vi "Check Status (No Objects).vi"(8 "error in (no error)":errorcluster, 11 "Cluster In":T3={"helium"={"fastHe?"=FALSE, "slowHe?"=FALSE, "fillHe?"=FALSE, "lowHe?"=FALSE}, "nitrogen"={"fillN?"=FALSE, "lowN?"=FALSE}, "Shutdown"=FALSE, "Cryogen Levels"=[], "IO Info"={"Address"={"Com Port"=1, "ISOBUS Address"=5, "GPIB Address"=24, "Communication"=enum."ISOBUS"}, "ILM Name"="", "Display Channel"=[]}} {"Cryogen Levels" min=-1.0 max=100.0 scale=0.0..100.0}) -> (0 "error out":errorcluster, 1 "Status":string, 2 "On?":bool, 3 "Cluster Out":T3={"helium"={"fastHe?"=FALSE, "slowHe?"=FALSE, "fillHe?"=FALSE, "lowHe?"=FALSE}, "nitrogen"={"fillN?"=FALSE, "lowN?"=FALSE}, "Shutdown"=FALSE, "Cryogen Levels"=[], "IO Info"={"Address"={"Com Port"=1, "ISOBUS Address"=5, "GPIB Address"=24, "Communication"=enum."ISOBUS"}, "ILM Name"="", "Display Channel"=[]}} {"Cryogen Levels" min=-1.0 max=100.0 scale=0.0..100.0})   [LabVIEW 2009]
uses:
  Cryogen Levels.ctl
  Oxford/BUSGEN.LLB/OxfordAddress.ctl
  Level Meter.lvclass
panel:
  out "cryolevels":T1 min=-1.0 max=100.0 scale=0.0..100.0
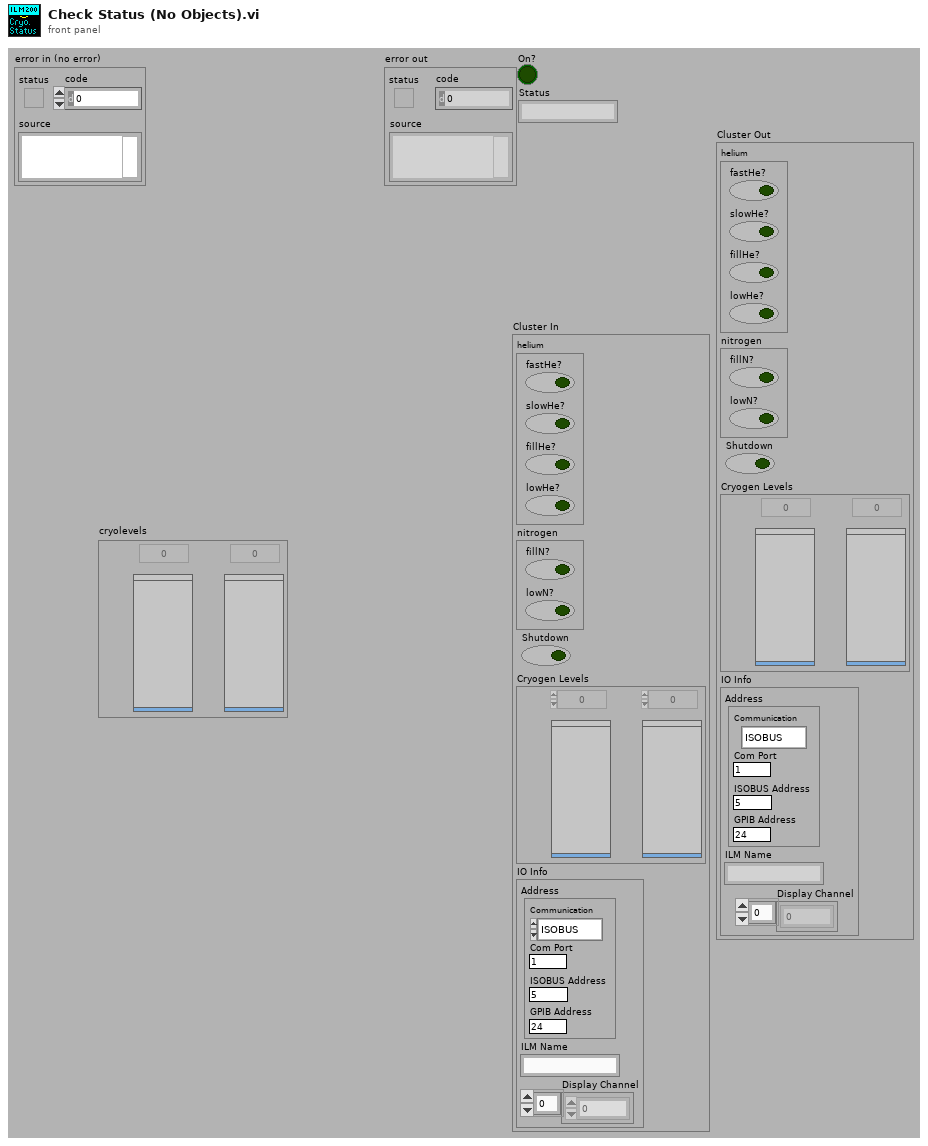
[diagram p1: front panel]
types:
  T1 = typedef "Level Meter.lvclass/Cryogen Levels.ctl" = dbl[]
  T2 = typedef "OxfordAddress.ctl" = cluster{"Com Port":i32, "ISOBUS Address":i32, "GPIB Address":i16, "Communication":enum16{"RS232", "ISOBUS", "GPIB", "Gateway"}}
  T3 = cluster{"helium":cluster{"fastHe?":bool, "slowHe?":bool, "fillHe?":bool, "lowHe?":bool}, "nitrogen":cluster{"fillN?":bool, "lowN?":bool}, "Shutdown":bool, "Cryogen Levels":T1, "IO Info":cluster{"Address":T2, "ILM Name":string, "Display Channel":i32[]}}
  T4 = typedef "Readable.lvclass/X array.ctl" = T5[]
  T5 = typedef "Readable.lvclass/X.ctl" = dbl
  T6 = typedef "ILMRelayStatus.ctl" = cluster{"Shut down":bool, "Alarm sound":bool, "Alarm state":bool, "Silence prohib":bool, "Relay1 active":bool, "Relay 2 active":bool, "Relay 3 active":bool, "Relay 4 active":bool}
  T7 = typedef "ILMChannelStatus.ctl" = cluster{"Probe current":bool, "Probe fast":bool, "Probe slow":bool, "Auto-fill":enum16{"End fill", "Not filling", "Filling", "Start filling"}, "Fill":bool, "Low level":bool, "Alm requested":bool, "Pre-pulse I":bool}
  T8 = cluster{bool, bool, "Fill":bool, "Low level":bool}
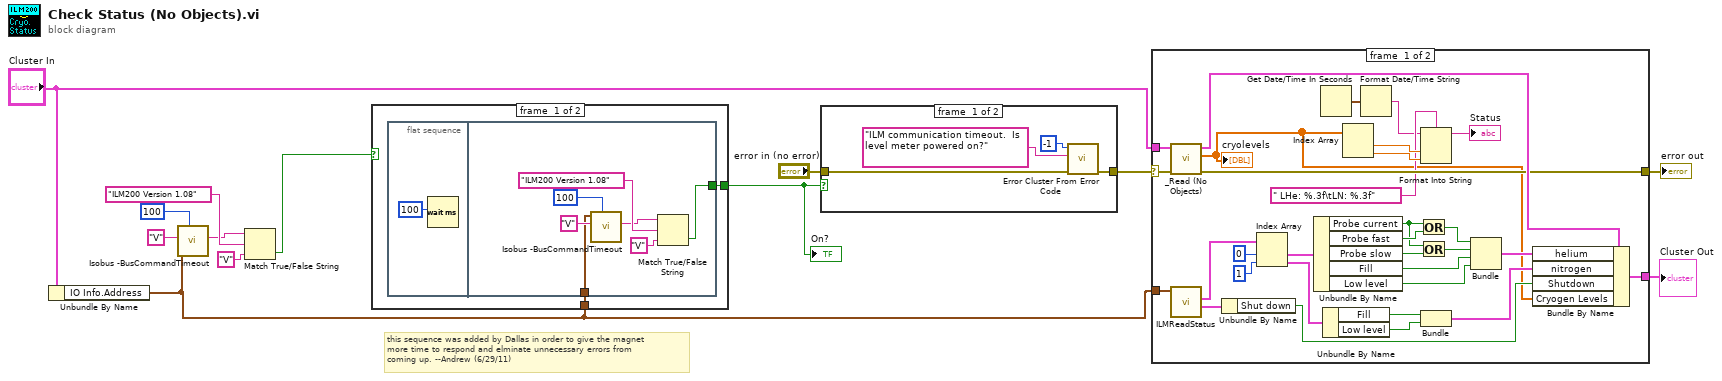
[diagram p0: block diagram]
diagram:
  # "this sequence was added by Dallas in order to give the magnet\nmore time to respond and elminate unnecessary errors from\ncoming up. --Andrew (6/29/11)"
  n1 = Unbundle By Name("Cluster In") -> ("IO Info.Address"=w5:T2)
  n2 = call "Isobus -BusCommandTimeout.vi"("Timeout (ms)"=100, "Command"="V", "Address"=w5) -> ("Reply"=w8:string)  [unwired: 5 out]
  n3 = Match True/False String(2:"V", 3:"ILM200 Version 1.08", 4:w8) -> (0:w3:bool)  [unwired: 1 out]
  n4 = case shown="False" w3 {
    selector: w3 -> [_ w24]
    tunnel: w5 -> [w15 _]
    tunnel: [w14 w24] -> w4
    frame #0 {
      n5 = flat-sequence {
        tunnel: w15 -> [w18]
        tunnel: [w17] -> w14
        frame #0 {
          n6 = Wait (ms)(milliseconds to wait=u32 100) -> ()  [unwired: 1 out]
        }
        frame #1 {
          n7 = call "Isobus -BusCommandTimeout.vi"("Timeout (ms)"=100, "Command"="V", "Address"=w18) -> ("Reply"=w19:string)  [unwired: 5 out]
          n8 = Match True/False String(2:"V", 3:"ILM200 Version 1.08", 4:w19) -> (0:w17:bool)  [unwired: 1 out]
        }
      }
    }
    frame #1 {
    }
  }
  "On?" <- w4
  n9 = case shown="False" w4 {
    tunnel: "error in (no error)" -> [w27 w29]
    tunnel: [w26 w29] -> w6
    frame #0 {
      n10 = call <vilib>:"Error Cluster From Error Code.vi"("error in (no error)"=w27, "error message (\"\")"="ILM communication timeout.  Is level meter powered on?" ("error message (\"\")"), "error code (0)"=-1) -> ("error out"=w26:errorcluster)  [unwired: 6 in]
    }
    frame #1 {
    }
  }
  n11 = case shown="No Error" w6 {
    selector: w6 -> [w33 w61]
    tunnel: [w45 w62] -> w1
    tunnel: [w40 w61] -> w13
    tunnel: "Cluster In" -> [w30 w62]
    tunnel: w5 -> [w34 _]
    frame #0 {
      n12 = call "_Read (No Objects).vi"("error in (no error)"=w33, "Cluster In"=w30) -> ("error out"=w40:errorcluster, "X array"=w35:T4, "Cluster Out"=w41:T3)  [unwired: 7 in]
      "cryolevels" <- w35
      n13 = call "ILMReadStatus.vi"("Instrument address"=w34) -> ("Relay"=w46:T6, "Channel"=w60:T7[])  [unwired: 5 out]
      n14 = Unbundle By Name(w46) -> ("Shut down"=w42:bool)
      n15 = Index Array(array=w60, index #1=0, index #2=1) -> (element #1=w57:T7, element #2=w56:T7)
      n16 = Unbundle By Name(w57) -> ("Probe current"=w53:bool, "Probe fast"=w54:bool, "Probe slow"=w55:bool, "Fill"=w49:bool, "Low level"=w51:bool)
      n17 = Get Date/Time In Seconds() -> (seconds since 1Jan1904=w31:timestamp)
      n18 = Unbundle By Name(w56) -> ("Fill"=w48:bool, "Low level"=w47:bool)
      n19 = Index Array(array=w35) -> (element #1=w39:T5, element #2=w38:T5)  [unwired: 2 in]
      n20 = Format Date/Time String(seconds (now)=w31) -> (date/time string=w32:string)  [unwired: 2 in]
      n21 = Or(x=w53, y=w54) -> (x .or. y?=w52:bool)
      n22 = Or(x=w53, y=w55) -> (x .or. y?=w50:bool)
      n23 = Format Into String(format string=" LHe: %.3f\tLN: %.3f", initial string=w32, w39, w38) -> (resulting string=→"Status":string)  [unwired: 1 in, 1 out]
      n24 = Bundle("Fill"=w48, "Low level"=w47) -> (w43:cluster{"Fill":bool, "Low level":bool})  [unwired: 1 out]
      n25 = Bundle(w52, w50, "Fill"=w49, "Low level"=w51) -> (w44:T8)  [unwired: 1 out]
      n26 = Bundle By Name(cluster=w41, "helium"=w44, "nitrogen"=w43, "Shutdown"=w42, "Cryogen Levels"=w35) -> (w45:T3)
    }
    frame #1 {
    }
  }
  "error out" <- w13
  "Cluster Out" <- w1
